vi "WFS Get Spot Intensities.vi"(8 "error in (no error)":errorcluster {"code" format="%.0x"}, 11 "instrument handle":refnum<visa-resource-name>) -> (0 "error out":errorcluster {"code" format="%.0x"}, 2 "Array Intensity":sgl[](array[numeric]) format="%.2p", 3 "instrument handle out":refnum<visa-resource-name>)   [LabVIEW 2020]
doc: "This VI returns a two-dimensional array containing the spot intensities in arbitrary unit calculated by WFS Calc Spots Centr Dia Intens.vi.\n\nNote: WFS Calc Spots Centr Dia Intens.vi is required to run successfully before calculated data can be retrieved."
uses:
  WFS_32.dll
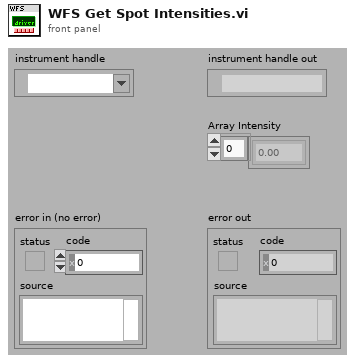
[diagram p1: front panel]
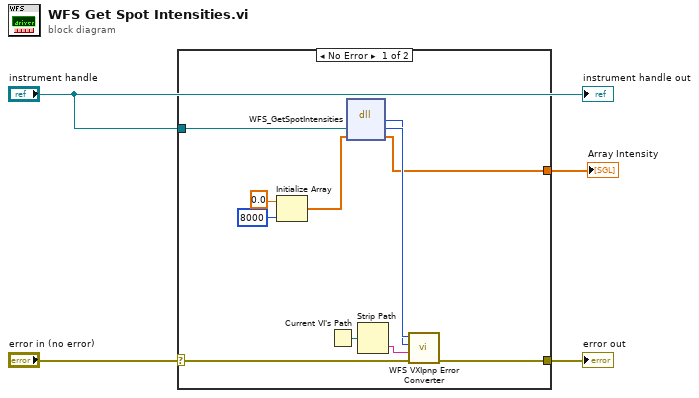
[diagram p0: block diagram]
diagram:
  n1 = case shown="No Error" "error in (no error)" {
    selector: "error in (no error)" -> [w10 w16]
    tunnel: [w9 w16] -> w4
    tunnel: "instrument handle" -> [w14 _]
    tunnel: [w5 _] -> w1
    frame No Error {
      n2 = Initialize Array(sgl 0.0 ("element"), 8000 ("dimension size")) -> (w8:sgl[])
      n3 = Current VI's Path() -> (path=w15:path)
      n4 = dll-call lib="WFS_*.*" fn="WFS_GetSpotIntensities"("Instrument Handle"=w14, "Array Intensity"=w8) -> (w12:i32, "Instrument Handle"=w13:u32, "Array Intensity"=w5:sgl[])  [unwired: 3 in, 2 out]
      n5 = Strip Path(path=w15) -> (name=w11:string)  [unwired: 1 out]
      n6 = call "WFS VXIpnp Error Converter.vi"("error in (no error)"=w10, "Name Of VI (\"\")"=w11, "CVI Error Code (0)"=w12, "instrument handle"=w13) -> ("error out"=w9:errorcluster)  [unwired: 6 in, 1 out]
    }
    frame Error {
    }
  }
  "error out" <- w4
  "Array Intensity" <- w1
  "instrument handle out" <- "instrument handle"
